vi "Add MeasLink Indicators.vi"(11 "error in (no error)":errorcluster) -> (15 "error out":errorcluster)   [LabVIEW 2021, in "Converter.lvlib"]
uses:
  Converter.lvlib
  Path Functions/Path Functions.lvlib
  Converter Reusables/Converter Reusables.lvlib
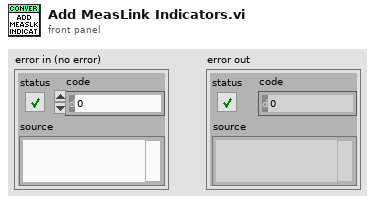
[diagram p1: front panel]
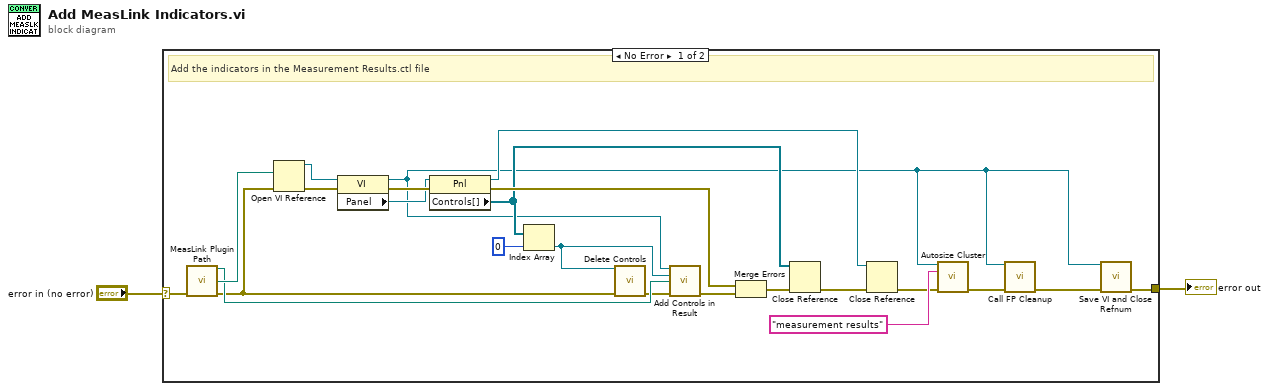
[diagram p0: block diagram]
diagram:
  n1 = case shown="No Error" "error in (no error)" {
    selector: "error in (no error)" -> [w14 w26]
    tunnel: [w18 w26] -> w2
    frame No Error {
      # "Add the indicators in the Measurement Results.ctl file"
      n2 = call "MeasLink Plugin Path.vi"("error in (no error)"=w14) -> ("New Code Module"=w6:path, "Result Control"=w15:path, "error out"=w3:errorcluster)  [unwired: 2 in, 10 out]
      n3 = Open VI Reference(vi path=w15, error in (no error)=w3) -> (vi reference=w8:refnum<vi>, error out=w21:errorcluster)  [unwired: 4 in]
      n4 = property class="VI"(reference=w8, error in=w21) -> (reference out=w7:refnum<vi>, error out=w25:errorcluster, "Panel"=w22:refnum<vi>)
      n5 = property class="Pnl"(reference=w22, error in=w25) -> (reference out=w13:refnum<vi>, error out=w12:errorcluster, "Controls[]"=w11:refnum<vi>[])
      n6 = Index Array(array=w11, index=0) -> (element=w5:refnum<vi>)
      n7 = call "Delete Controls.vi"("Control in"=w5, "error in (no error)"=w3) -> ("error out"=w4:errorcluster)  [unwired: 13 in]
      n8 = call "Add Controls in Result.vi"("VI Reference"=w7, "Result Cluster"=w5, "New Code Module"=w6, "error in (no error)"=w4) -> ("error out"=w23:errorcluster)  [unwired: 11 in]
      n9 = Merge Errors(w12, w23) -> (w10:errorcluster)
      n10 = Close Reference(reference=w11, error in (no error)=w10) -> (error out=w9:errorcluster)
      n11 = Close Reference(reference=w13, error in (no error)=w9) -> (error out=w19:errorcluster)
      n12 = call "Autosize Cluster.vi"("VI Refnum"=w7, "name"="measurement results" ("name/order"), "error in (no error)"=w19) -> ("error out"=w17:errorcluster)  [unwired: 12 in]
      n13 = call "Call FP Cleanup.vi"("VI"=w7, "error in (no error)"=w17) -> ("error out"=w16:errorcluster)  [unwired: 13 in]
      n14 = call "Save VI and Close Refnum.vi"("VI Refnum"=w7, "error in"=w16) -> ("error out"=w18:errorcluster)  [unwired: 13 in]
    }
    frame Error {
    }
  }
  "error out" <- w2
